vi "round a number.vi"(10 "# decimal places to keep":i32, 11 "Raw Value":dbl format="%.4f") -> (3 "Rounded Value":dbl format="%.4f")   [LabVIEW 2021]
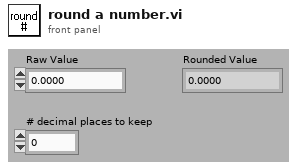
[diagram p1: front panel]
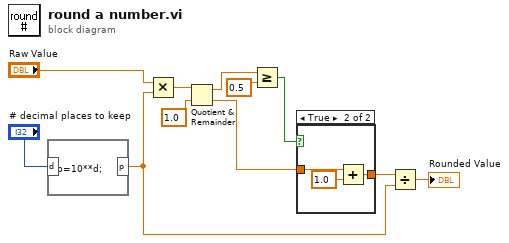
[diagram p0: block diagram]
diagram:
  n1 = formula code="p=10**d;"("d"="# decimal places to keep") -> ("p"=w1:dbl)
  n2 = Multiply(x="Raw Value", y=w1) -> (x*y=w10:dbl)
  n3 = Quotient & Remainder(x=w10, y=1.0) -> (x-y*floor(x/y)=w8:dbl, floor(x/y)=w5:dbl)
  n4 = Greater Or Equal?(x=w8, y=0.5) -> (x >= y?=w6:bool)
  n5 = case shown="True" w6 {
    tunnel: w5 -> [w12 w15]
    tunnel: [w12 w13] -> w4
    frame False {
    }
    frame True {
      n6 = Add(x=w15, y=1.0) -> (x+y=w13:dbl)
    }
  }
  n7 = Divide(x=w4, y=w1) -> (x/y=→"Rounded Value":dbl)
